vi "ArenaVisualDebugger2017.vi"() -> ()   [LabVIEW 2015, in "MissionControl2017.lvlib" / "DebuggingTools.lvlib"]
uses:
  DebuggingTools.lvlib
  PathfindingSettings.ctl
  MovementSettings.ctl
  PathCostWeights.ctl
  IntermediatePositionGrids.ctl
  <vilib>/Utility/miscctls.llb/LVPoint32TypeDef.ctl
  LocalizationStatus.ctl
  <vilib>/Utility/miscctls.llb/LVBoundsTypeDef.ctl
  Vector.ctl
  Move.ctl
  PathOfMoves.ctl
  Overlord2017.lvlib
  SubVIs - MissionControl2017.lvlib
  TestbenchUtils - Navigation2017.lvlib
  Types - Navigation2017.lvlib
  Navigation2017.lvlib
  SubVIs - Navigation2017.lvlib
panel:
  out "Total Paths Arrived":dbl=484.0
  in  "WaitingForLocalization":bool=TRUE
  in  "Pathfind Turning Radius (m)":dbl(knob)=2.5661842935373853 scale=0.0..4.0
  in  "reset timer":bool
  out "millisecond timer value":u32=9071
  in  "Movement Control Turn Tightness":dbl(slide)=6.226706181197886 scale=1.0..10.0
  out "Right Motor PWM":dbl(graph)
  out "Left Motor PWM":dbl(graph)
  out "Motor PWM XY Graph":cluster{"X":dbl, "Y":dbl}[](graph)
  out "Position at Start of Pathfinding Calculation":T1
  out "Current Localization Status (As Drawn Above)":T1={"x"=4.84866, "y"=1.21078125, "angle"=-2.748893571891069, "valid"=TRUE, "lastUpdatedTime"=858082015.0}
  in  "Debug Mining":bool=TRUE
  in  "Debug Wheel Motors":bool=TRUE
  out "navDebugBotSpin":dbl=-2.748893571891069
  out "y (m)":dbl=0.0221484375
  out "x (m)":dbl=5.26932
  in  "Debug Localization - Mouse":bool=TRUE
  out "Mouse Wheel Sum":dbl=-1.0
  out "Mouse Wheel Delta":i32=-1
  out "Mouse Down Button":u16=1
  out "Mouse Coords":T2={"Horizontal"=286, "Vertical"=3}
  out "Mouse Down Coords":T2={"Horizontal"=343, "Vertical"=164}
  out "CurrMiningRun":i16(slide) scale=0.0..3.0
  out "CurrStage":string
  out "UsedDesperation":bool
  out "SpecifyingEndAngle":bool=TRUE
  out "NextPointIsDestination":bool
  out "CurrNavStage":string
  out "FPS Indicator":bool
  in  "Pathfinding Settings":T3={"Movement Settings"={"Arrival Tolerance (m)"=0.01, "Closeness Threshold (m)"=0.5, "Pit Obstacle Radius (m)"=0.5, "Pit Locations"=[]}, "Dead Zone"=0.85, "Max Moves"=4.0, "Move Segment Length (m)"=0.2, "Path Cost Weights"={"Length Weight"=1.0, "Angle Weight"=0.0, "Angle Error Weight"=1000.0, "Angle Error Threshold"=0.314, "Per Move Penalty"=0.05, "Closeness Weight"=100.0, "Too Short Penalty"=100.0, "Too Short Threshold"=1.5}, "Desperation - Reduction Per Attempt (Ratio)"=0.9, "Desperation - Max Attempts"=1, "Log All Move Points"=TRUE, "Intermediate Position Grids"=[{"x1"=0.0, "x2"=1.75, "resolution"=0.4}, {"x1"=1.75, "x2"=4.5, "resolution"=0.4}]}
  out "Arena Pixel Size":i16[](array[numeric])=[1000, 512]
  out "Arena Control":picture
  # "NOTE: Open and pin\n\nMineOrDumpBlocking.vi\nand\nSetWheelMotorPWM.vi\n\nalongside when debugging."
  # "(Spin robot with arrow keys)"
  # "To toggle localization debugging:\n- Flip this switch <---\n- Set the Project Property -> Conditional Compilation Property\n\"DISCONNECT_LOCALIZATION\" to True or False"
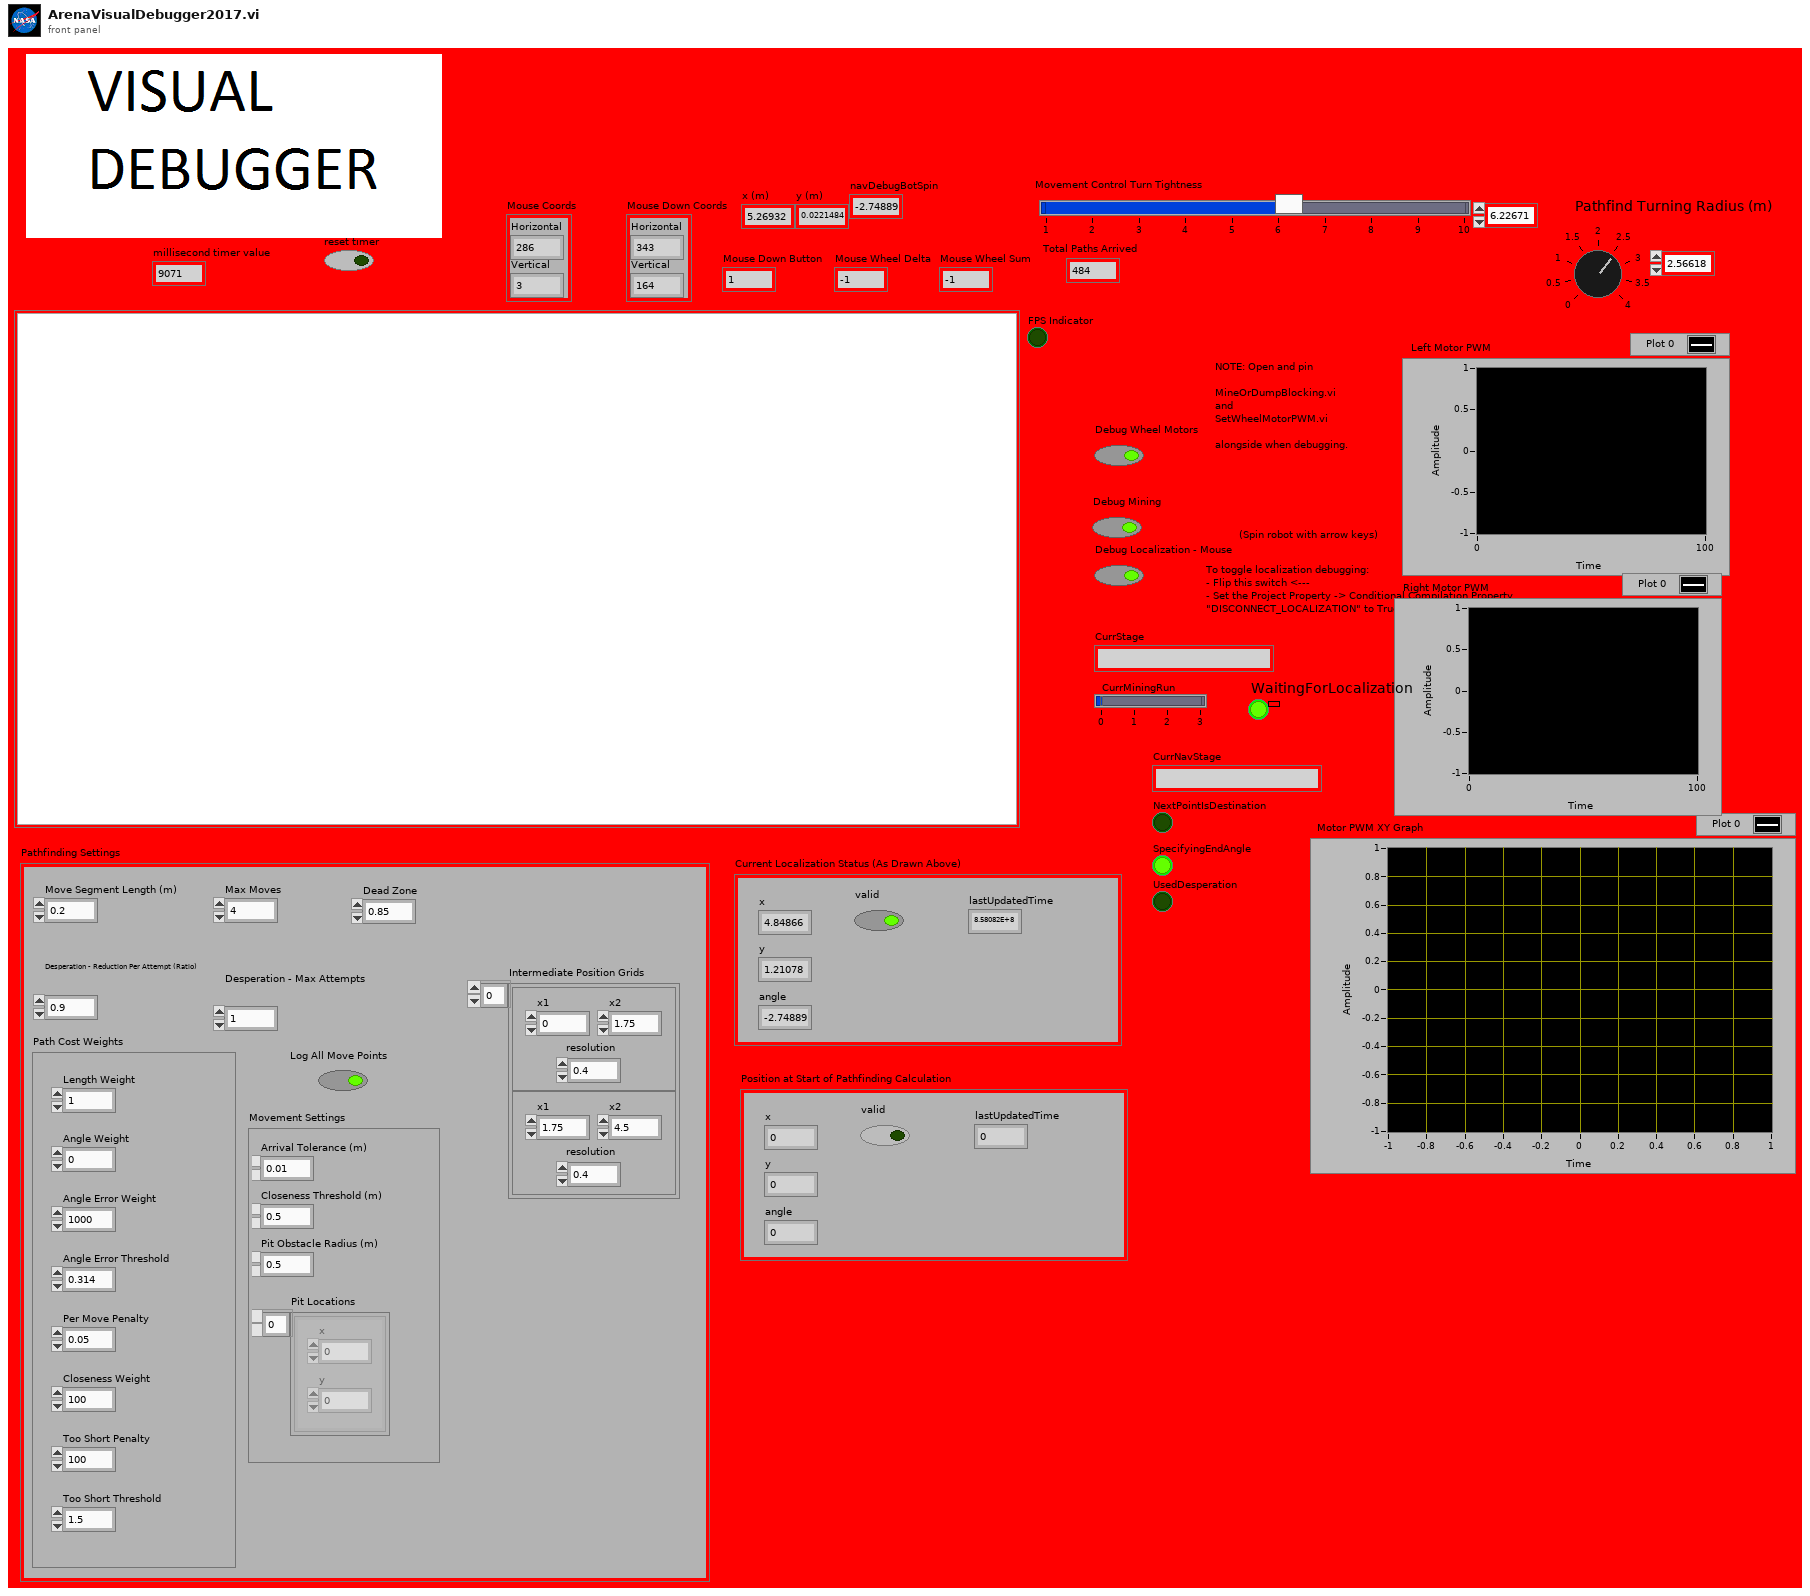
[diagram p1: front panel]
types:
  T1 = typedef "Navigation2017.lvlib/TestbenchUtils - Navigation2017.lvlib/LocalizationStatus.ctl" = cluster{"x":dbl, "y":dbl, "angle":dbl, "valid":bool, "lastUpdatedTime":dbl}
  T2 = typedef "LVPoint32TypeDef.ctl" = cluster{"Horizontal":i32, "Vertical":i32}
  T3 = typedef "Navigation2017.lvlib/Types - Navigation2017.lvlib/PathfindingSettings.ctl" = cluster{"Movement Settings":T4, "Dead Zone":dbl, "Max Moves":dbl, "Move Segment Length (m)":dbl, "Path Cost Weights":T5, "Desperation - Reduction Per Attempt (Ratio)":dbl, "Desperation - Max Attempts":i16, "Log All Move Points":bool, "Intermediate Position Grids":T6}
  T4 = typedef "Navigation2017.lvlib/Types - Navigation2017.lvlib/MovementSettings.ctl" = cluster{"Arrival Tolerance (m)":dbl, "Closeness Threshold (m)":dbl, "Pit Obstacle Radius (m)":dbl, "Pit Locations":cluster{"x":dbl, "y":dbl}[]}
  T5 = typedef "Navigation2017.lvlib/Types - Navigation2017.lvlib/PathCostWeights.ctl" = cluster{"Length Weight":dbl, "Angle Weight":dbl, "Angle Error Weight":dbl, "Angle Error Threshold":dbl, "Per Move Penalty":dbl, "Closeness Weight":dbl, "Too Short Penalty":dbl, "Too Short Threshold":dbl}
  T6 = typedef "Navigation2017.lvlib/Types - Navigation2017.lvlib/IntermediatePositionGrids.ctl" = cluster{"x1":dbl, "x2":dbl, "resolution":dbl}[]
  T7 = typedef "LVBoundsTypeDef.ctl" = cluster{"Width":u32, "Height":u32}
  T8 = typedef "eventvkey.ctl" = enum16{"ASCII", "Enter", "Return", "Shift", "Ctrl", "Alt", "Cmd", "Opt", "Caps", "NumLock", "Clear", "Break", "Up", "Down", "Left", "Right", "Insert", "Delete", "Home", "End", "PageUp", "PageDown", "Escape", "Help", "Pause", "ScrollLock", "F1", "F2", "F3", "F4", "F5", "F6", "F7", "F8", "F9", "F10", "F11", "F12", "F13", "F14", "F15", "F16", "F17", "F18", "F19", "F20", "F21", "F22", "F23", "F24", "Play", "VolumeUp", "VolumeDown", "Mute", "Two Byte Char"}
  T9 = typedef "imagedata.ctl" = cluster{"image type":i32, "image depth":i32, "image":u8[], "mask":u8[], "colors":u32[], "Rectangle":cluster{"left":i16, "top":i16, "right":i16, "bottom":i16}}
  T10 = typedef "Navigation2017.lvlib/Types - Navigation2017.lvlib/Vector.ctl" = cluster{"x":dbl, "y":dbl, "angle":dbl}
  T11 = cluster{"Width":u16, "Style":enum32{"Solid", "Dash", "Dot", "DashDot", "DashDotDot"}}
  T12 = typedef "Navigation2017.lvlib/Types - Navigation2017.lvlib/PathOfMoves.ctl" = cluster{"Dest Angle Error":dbl, "Dest Angle Considered":bool, "Moves":T13[]}
  T13 = typedef "Navigation2017.lvlib/Types - Navigation2017.lvlib/Move.ctl" = cluster{"Did Reach Dest":bool, "Did Collide":bool, "Sum of Angle Changes (rad)":dbl, "Move Length (m)":dbl, "Closeness Sum":dbl, "Positions Along Move":T10[], "Moved Fwd":bool}
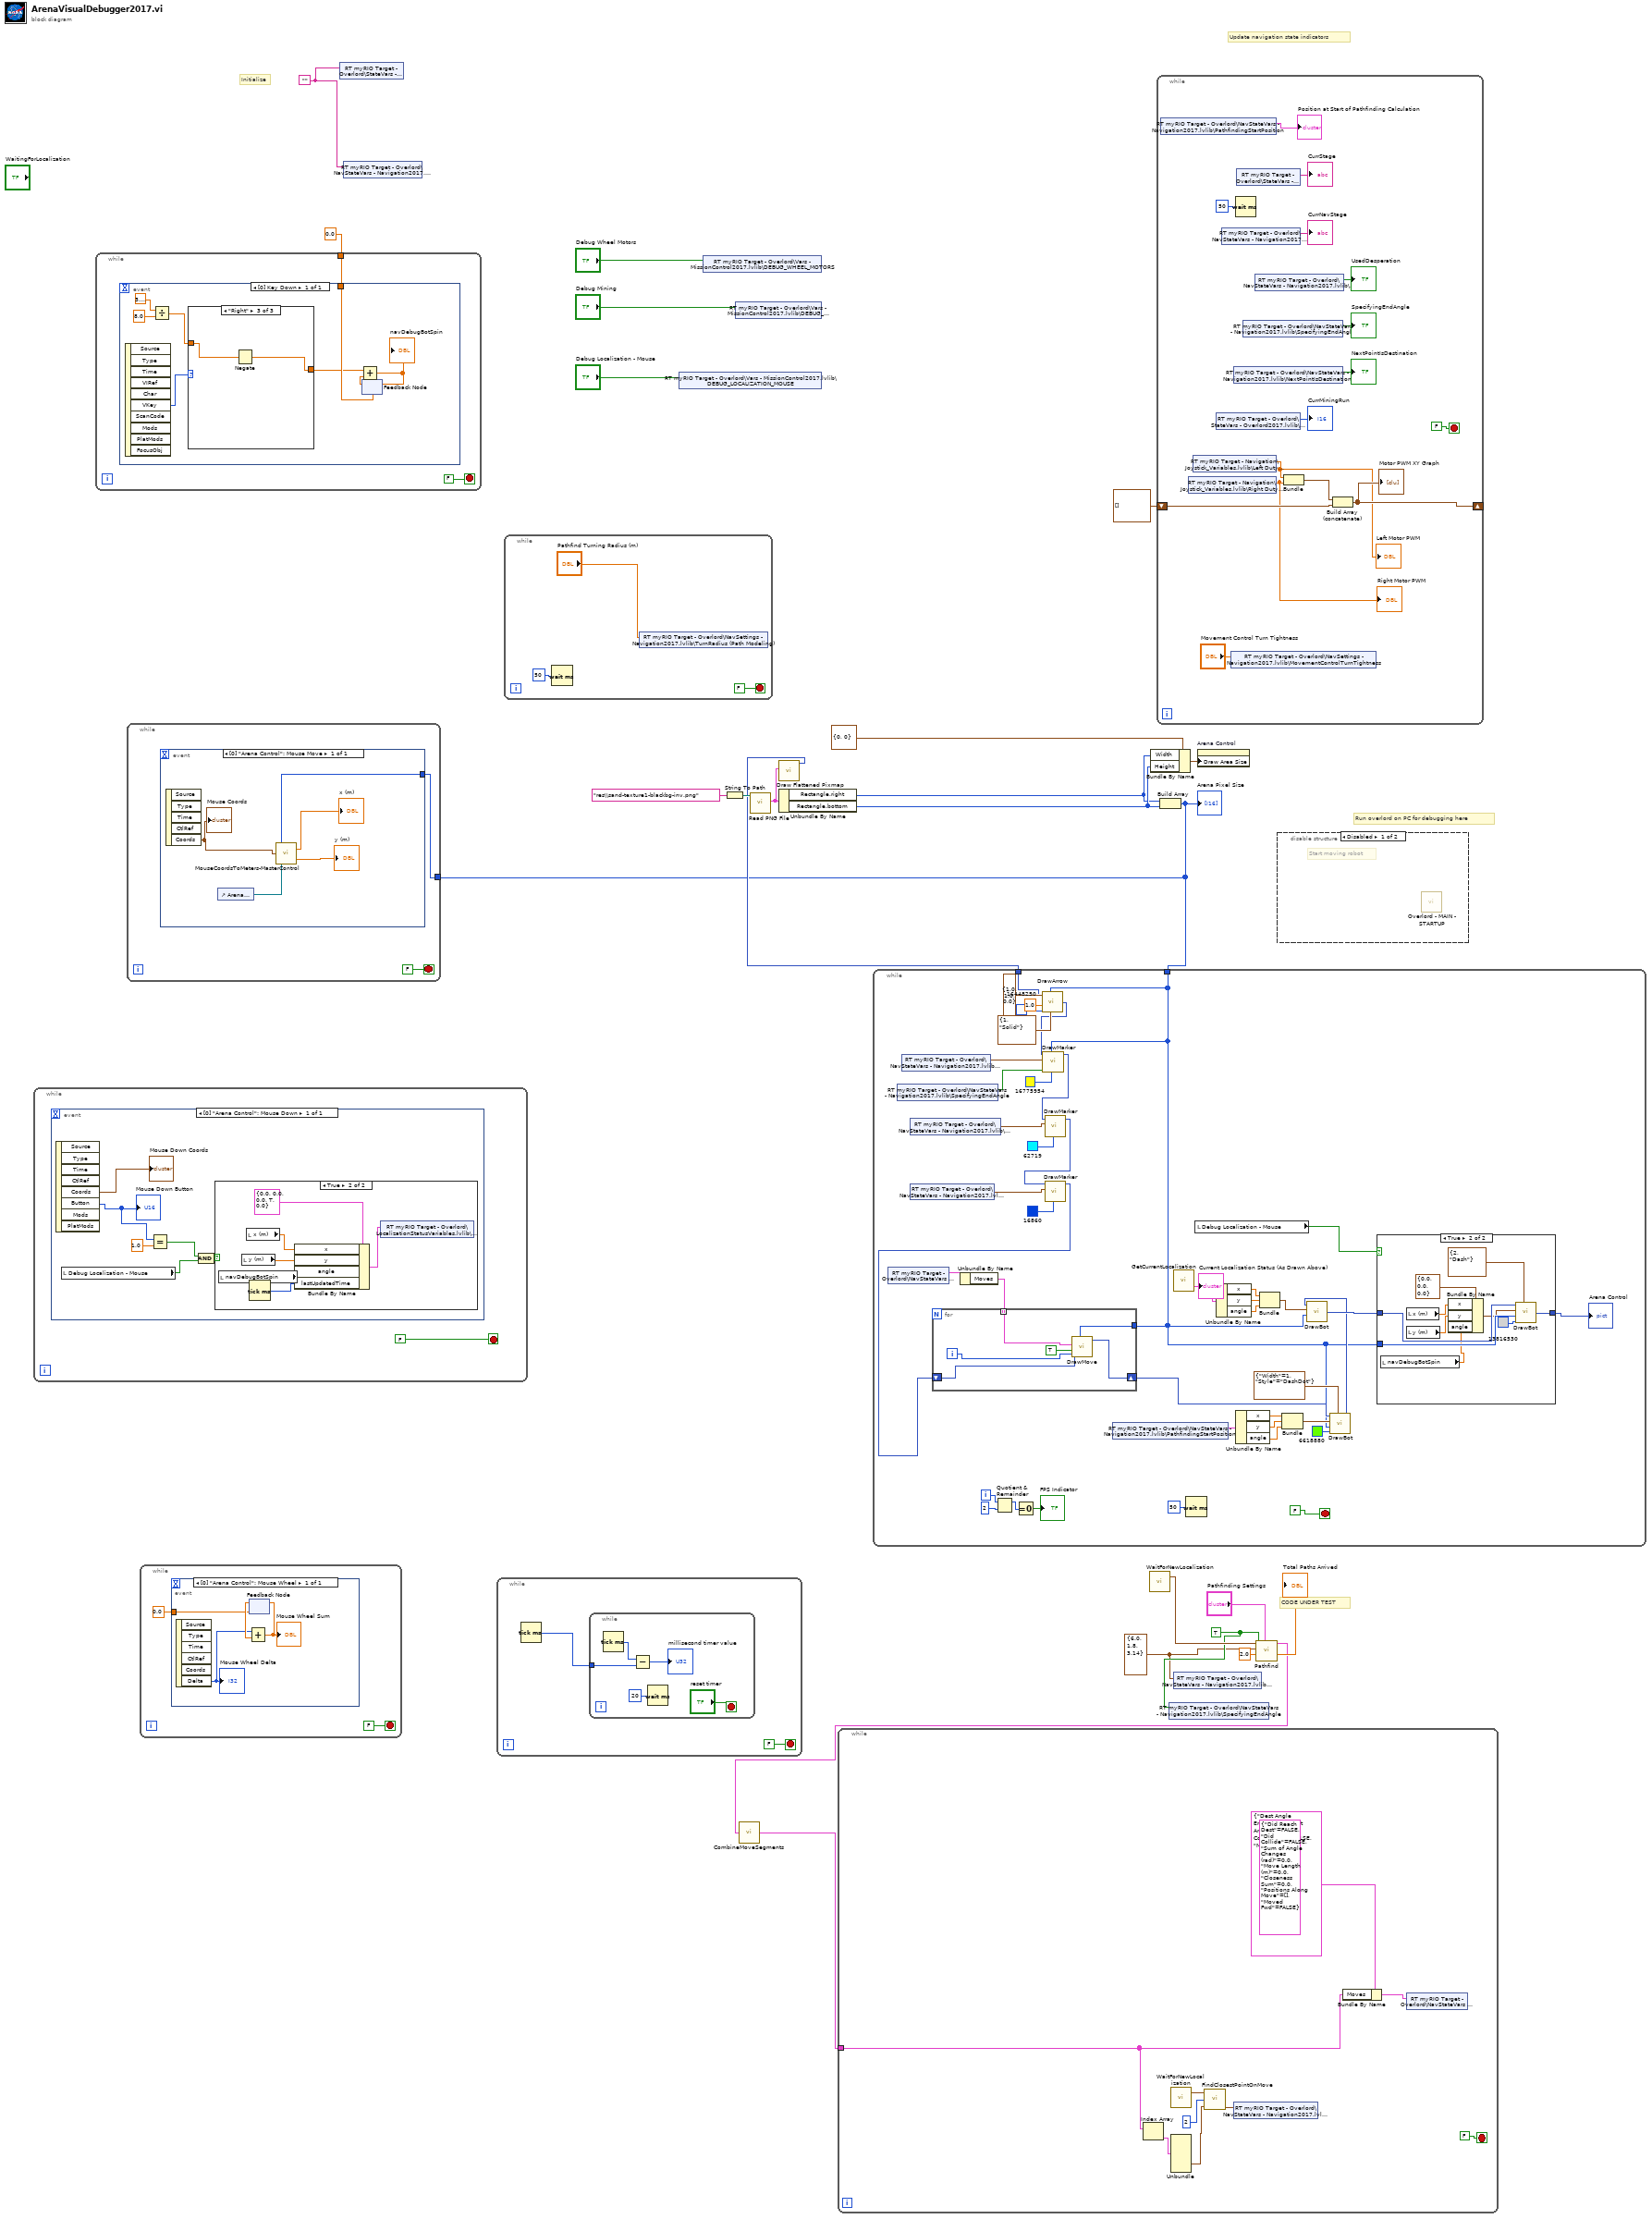
[diagram p0: block diagram]
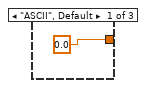
[diagram p3: hidden frame]
diagram:
  w5 = TRUE ("Specified End Angle")
  w4 = cluster{"x":dbl, "y":dbl, "angle":dbl} {"x"=6.0, "y"=1.8, "angle"=3.14} ("Destination")
  w13 = ""
  # "CODE UNDER TEST"
  # "Run overlord on PC for debugging here"
  # "Initialize"
  # "Update navigation state indicators"
  n1 = while {
    stop <- FALSE stop-if-true
    n2 = event shown="[0] \"Arena Control\": Mouse Down" {
      selector: _ -> [_]
      dyn-events: _ -> [_]
      timeout: _ -> [_]
      event "Arena Control": Mouse Down {
        n3 = event-data() -> ("Coords"=→"Mouse Down Coords":T2, "Button"=w28:u16)  [unwired: 1 in, 6 out]
        "Mouse Down Button" <- w28
        n4 = local read "Debug Localization - Mouse"() -> (w27:bool)
        n5 = Equal?(x=w28, y=1.0) -> (x = y?=w26:bool)
        n6 = And(x=w26, y=w27) -> (x .and. y?=w25:bool)
        n7 = case shown="True" w25 {
          frame False {
          }
          frame True {
            n8 = local read "navDebugBotSpin"() -> (w31:dbl)
            n9 = local read "y (m)"() -> (w32:dbl)
            n10 = local read "x (m)"() -> (w33:dbl)
            n11 = Tick Count (ms)() -> (millisecond timer value=w34:u32)
            n12 = Bundle By Name(cluster=T1 {"x"=0.0, "y"=0.0, "angle"=0.0, "valid"=TRUE, "lastUpdatedTime"=0.0} ("Localization Status"), "x"=w33, "y"=w32, "angle"=w31, "lastUpdatedTime"=w34) -> (w35:T1)
            n13 = shared-variable "RT myRIO Target - Overlord\\LocalizationStatusVariables.lvlib\\LocalizationStatus"(w35) -> ()  [unwired: 1 in, 1 out]
          }
        }
      }
    }
  }
  n14 = while {
    tunnel: 0.0 -> [w37]
    stop <- FALSE stop-if-true
    n15 = event shown="[0] Key Down" {
      selector: _ -> [_]
      dyn-events: _ -> [_]
      timeout: _ -> [_]
      tunnel: w37 -> [w43]
      event Key Down {
        n16 = event-data() -> ("VKey"=w46:T8)  [unwired: 1 in, 9 out]
        n17 = Divide(x=3.141592653589793, y=8.0) -> (x/y=w39:dbl)
        n18 = case shown="\"Right\"" w46 {
          tunnel: [0.0 w48 w49] -> w42
          tunnel: w39 -> [_ w48 w50]
          frame "ASCII", Default {
          }
          frame "Left" {
          }
          frame "Right" {
            n19 = Negate(x=w50) -> (-x=w49:dbl)
          }
        }
        n20 = feedback #1(w43) -> (w44:dbl)
        n21 = Add(x=w42, y=w44) -> (x+y=w45:dbl)
        "navDebugBotSpin" <- w45
        n22 = feedback-in #1(w45) -> ()
      }
    }
  }
  n23 = while {
    stop <- FALSE stop-if-true
    n24 = event shown="[0] \"Arena Control\": Mouse Wheel" {
      selector: _ -> [_]
      dyn-events: _ -> [_]
      timeout: _ -> [_]
      tunnel: 0.0 -> [w54]
      event "Arena Control": Mouse Wheel {
        n25 = event-data() -> ("Delta"=w53:i32)  [unwired: 1 in, 5 out]
        "Mouse Wheel Delta" <- w53
        n26 = feedback #2(w54) -> (w55:dbl)
        n27 = Add(x=w53, y=w55) -> (x+y=w56:dbl)
        "Mouse Wheel Sum" <- w56
        n28 = feedback-in #2(w56) -> ()
      }
    }
  }
  n29 = shared-variable "RT myRIO Target - Overlord\\StateVars - Overlord2017.lvlib\\CurrStage"(w13) -> ()  [unwired: 1 in, 1 out]
  n30 = shared-variable "RT myRIO Target - Overlord\\NavStateVars - Navigation2017.lvlib\\CurrNavStage"(w13) -> ()  [unwired: 1 in, 1 out]
  n31 = while {
    stop <- FALSE stop-if-true
    n32 = Tick Count (ms)() -> (millisecond timer value=w58:u32)
    n33 = while {
      tunnel: w58 -> [w60]
      stop <- "reset timer" stop-if-true
      n34 = Tick Count (ms)() -> (millisecond timer value=w61:u32)
      n35 = Subtract(x=w61, y=w60) -> (x-y=→"millisecond timer value":u32)
      n36 = Wait (ms)(milliseconds to wait=u32 20) -> ()  [unwired: 1 out]
    }
  }
  n37 = while {
    stop <- FALSE stop-if-true
    n38 = Wait (ms)(milliseconds to wait=u32 50) -> ()  [unwired: 1 out]
    n39 = shared-variable "RT myRIO Target - Overlord\\NavSettings - Navigation2017.lvlib\\TurnRadius (Path Modeling)"("Pathfind Turning Radius (m)") -> ()  [unwired: 1 in, 1 out]
  }
  n40 = shared-variable "RT myRIO Target - Overlord\\Vars - MissionControl2017.lvlib\\DEBUG_LOCALIZATION_MOUSE"("Debug Localization - Mouse") -> ()  [unwired: 1 in, 1 out]
  n41 = shared-variable "RT myRIO Target - Overlord\\Vars - MissionControl2017.lvlib\\DEBUG_WHEEL_MOTORS"("Debug Wheel Motors") -> ()  [unwired: 1 in, 1 out]
  n42 = String To Path(string="res\\sand-texture1-blackbg-inv.png" ("name or relative path")) -> (path=w22:path)
  n43 = shared-variable "RT myRIO Target - Overlord\\Vars - MissionControl2017.lvlib\\DEBUG_BUCKET"("Debug Mining") -> ()  [unwired: 1 in, 1 out]
  n44 = call <vilib>:"Read PNG File.vi"("path to PNG file"=w22) -> ("image data"=w17:T9)  [unwired: 8 in, 2 out]
  n45 = call <vilib>:"Draw Flattened Pixmap.vi"("image data"=w17) -> ("new picture"=w16:picture)  [unwired: 8 in]
  n46 = Unbundle By Name(w17) -> ("Rectangle.right"=w19:i16, "Rectangle.bottom"=w20:i16)
  n47 = call "WaitForNewLocalization.vi"() -> ("Localization Status Vector"=w6:T10)  [unwired: 1 out]
  n48 = Bundle By Name(cluster=T7 {"Width"=0, "Height"=0} ("Draw Area Size"), "Width"=w19, "Height"=w20) -> (w21:T7)
  n49 = while {
    shift-right: [w70] -> _
    shift-left: cluster{"Double":dbl, "Double":dbl}[] [] -> [w71]
    stop <- FALSE stop-if-true
    n50 = shared-variable "RT myRIO Target - Overlord\\NavStateVars - Navigation2017.lvlib\\PathfindingStartPosition"() -> (→"Position at Start of Pathfinding Calculation":T1)  [unwired: 1 in, 1 out]
    n51 = shared-variable "RT myRIO Target - Navigation\\Joystick_Variables.lvlib\\Right Duty Cycle"() -> (w69:dbl)  [unwired: 1 in, 1 out]
    "Right Motor PWM" <- w69
    n52 = shared-variable "RT myRIO Target - Navigation\\Joystick_Variables.lvlib\\Left Duty Cycle"() -> (w68:dbl)  [unwired: 1 in, 1 out]
    "Left Motor PWM" <- w68
    n53 = shared-variable "RT myRIO Target - Overlord\\StateVars - Overlord2017.lvlib\\CurrMiningRun"() -> (→"CurrMiningRun":i16)  [unwired: 1 in, 1 out]
    n54 = shared-variable "RT myRIO Target - Overlord\\NavStateVars - Navigation2017.lvlib\\CurrNavStage"() -> (→"CurrNavStage":string)  [unwired: 1 in, 1 out]
    n55 = shared-variable "RT myRIO Target - Overlord\\NavSettings - Navigation2017.lvlib\\MovementControlTurnTightness"("Movement Control Turn Tightness") -> ()  [unwired: 1 in, 1 out]
    n56 = shared-variable "RT myRIO Target - Overlord\\NavStateVars - Navigation2017.lvlib\\NextPointIsDestination"() -> (→"NextPointIsDestination":bool)  [unwired: 1 in, 1 out]
    n57 = Wait (ms)(milliseconds to wait=u32 50) -> ()  [unwired: 1 out]
    n58 = shared-variable "RT myRIO Target - Overlord\\StateVars - Overlord2017.lvlib\\CurrStage"() -> (→"CurrStage":string)  [unwired: 1 in, 1 out]
    n59 = shared-variable "RT myRIO Target - Overlord\\NavStateVars - Navigation2017.lvlib\\SpecifyingEndAngle"() -> (→"SpecifyingEndAngle":bool)  [unwired: 1 in, 1 out]
    n60 = shared-variable "RT myRIO Target - Overlord\\NavStateVars - Navigation2017.lvlib\\UsedDesperation"() -> (→"UsedDesperation":bool)  [unwired: 1 in, 1 out]
    n61 = Bundle("Double"=w68, "Double"=w69) -> (w72:cluster{"Double":dbl, "Double":dbl})  [unwired: 1 in]
    n62 = Build Array (concatenate)(w72, w71) -> (w70:cluster{"Double":dbl, "Double":dbl}[])
    "Motor PWM XY Graph" <- w70
  }
  n63 = Build Array(w19, w20) -> (w14:i16[])
  "Arena Pixel Size" <- w14
  n64 = while {
    tunnel: w14 -> [w82]
    stop <- FALSE stop-if-true
    n65 = event shown="[0] \"Arena Control\": Mouse Move" {
      selector: _ -> [_]
      dyn-events: _ -> [_]
      timeout: _ -> [_]
      tunnel: w82 -> [w87]
      event "Arena Control": Mouse Move {
        n66 = event-data() -> ("Coords"=w88:T2)  [unwired: 1 in, 4 out]
        "Mouse Coords" <- w88
        n67 = control-ref of="Arena Control"() -> (w86:refnum<vi>)
        n68 = call "MouseCoordsToMeters-MasterControl.vi"("Picture Control Ref"=w86, "Mouse Pos"=w88, "Arena Pixel Dim"=w87) -> ("y (m)"=→"y (m)":dbl, "x (m)"=→"x (m)":dbl)
      }
    }
  }
  n69 = while {
    tunnel: w16 -> [w91]
    tunnel: w14 -> [w90]
    i -> [w129]
    stop <- FALSE stop-if-true
    n70 = shared-variable "RT myRIO Target - Overlord\\NavStateVars - Navigation2017.lvlib\\CurrPath"() -> (w117:T12)  [unwired: 1 in, 1 out]
    n71 = shared-variable "RT myRIO Target - Overlord\\NavStateVars - Navigation2017.lvlib\\SpecifyingEndAngle"() -> (w109:bool)  [unwired: 1 in, 1 out]
    n72 = shared-variable "RT myRIO Target - Overlord\\NavStateVars - Navigation2017.lvlib\\DestinationPoint"() -> (w110:T10)  [unwired: 1 in, 1 out]
    n73 = shared-variable "RT myRIO Target - Overlord\\NavStateVars - Navigation2017.lvlib\\NextPointOnPath"() -> (w111:T10)  [unwired: 1 in, 1 out]
    n74 = shared-variable "RT myRIO Target - Overlord\\NavStateVars - Navigation2017.lvlib\\CurrPosOnPath"() -> (w99:T10)  [unwired: 1 in, 1 out]
    n75 = Unbundle By Name(w117) -> ("Moves"=w116:T13[])
    n76 = Quotient & Remainder(x=w129, y=2) -> (x-y*floor(x/y)=w120:i32)  [unwired: 1 out]
    n77 = Equal To 0?(x=w120) -> (x = 0?=→"FPS Indicator":bool)
    n78 = call "DrawArrow.vi"("Pen Style"=T11 {"Width"=1, "Style"=enum."Solid"}, "Arena Pixel Dim"=w90, "Color"=u32 16448250, "Length (m)"=1.0, "Vector (m)"=T10 {"x"=1.0, "y"=1.0, "angle"=0.0}, "picture"=w91) -> ("new picture"=w89:picture)
    n79 = call "DrawMarker.vi"("color(black)"=u32 16775954, "Arena Pixel Dim"=w90, "Draw An Arrow"=w109, "Cluster"=w110, "picture in"=w89) -> ("new picture"=w115:picture)  [unwired: 6 in]
    n80 = call "DrawMarker.vi"("color(black)"=u32 62719, "Cluster"=w111, "picture in"=w115) -> ("new picture"=w97:picture)  [unwired: 8 in]
    n81 = call "DrawMarker.vi"("color(black)"=u32 16860, "Cluster"=w99, "picture in"=w97) -> ("new picture"=w96:picture)  [unwired: 8 in]
    n82 = for {
      tunnel: w90 -> [w134]
      shift-right: [w135] -> w108
      shift-left: w96 -> [w136]
      tunnel: w116 -> [w132] mode=indexing
      i -> [w131]
      n83 = call "DrawMove.vi"("Arena Pixel Dim"=w134, "Move Number (optional)"=w131, "Show Vectors?"=TRUE, "Move"=w132, "picture in"=w136) -> ("picture out"=w135:picture)  [unwired: 3 in]
    }
    n84 = shared-variable "RT myRIO Target - Overlord\\NavStateVars - Navigation2017.lvlib\\PathfindingStartPosition"() -> (w103:T1)  [unwired: 1 in, 1 out]
    n85 = call "GetCurrentLocalization.vi"() -> ("Current Localization Status"=w122:T1)  [unwired: 1 out]
    "Current Localization Status (As Drawn Above)" <- w122
    n86 = Wait (ms)(milliseconds to wait=u32 50) -> ()  [unwired: 1 out]
    n87 = local read "Debug Localization - Mouse"() -> (w112:bool)
    n88 = Unbundle By Name(w122) -> ("x"=w125:dbl, "y"=w124:dbl, "angle"=w123:dbl)
    n89 = Unbundle By Name(w103) -> ("x"=w102:dbl, "y"=w101:dbl, "angle"=w100:dbl)
    n90 = Bundle("x"=w125, "y"=w124, "angle"=w123) -> (w121:cluster{"x":dbl, "y":dbl, "angle":dbl})  [unwired: 1 in]
    n91 = Bundle("x"=w102, "y"=w101, "angle"=w100) -> (w104:cluster{"x":dbl, "y":dbl, "angle":dbl})  [unwired: 1 in]
    n92 = call "DrawBot.vi"("picture in"=w108, "bot pos vector"=w104, "Arena Pixel Size"=w90, "bot color"=u32 6618880, "pen"=T11 {"Width"=1, "Style"=enum."DashDot"}) -> ("picture out"=w107:picture)
    n93 = call "DrawBot.vi"("picture in"=w107, "bot pos vector"=w121, "Arena Pixel Size"=w90) -> ("picture out"=w119:picture)  [unwired: 2 in]
    n94 = case shown="True" w112 {
      tunnel: w119 -> [w137 w147]
      tunnel: [w137 w146] -> w118
      tunnel: w90 -> [_ w143]
      frame False {
      }
      frame True {
        n95 = local read "navDebugBotSpin"() -> (w138:dbl)
        n96 = local read "x (m)"() -> (w140:dbl)
        n97 = local read "y (m)"() -> (w141:dbl)
        n98 = Bundle By Name(cluster=T10 {"x"=0.0, "y"=0.0, "angle"=0.0} ("Vector"), "x"=w140, "y"=w141, "angle"=w138) -> (w142:T10)
        n99 = call "DrawBot.vi"("picture in"=w147, "bot pos vector"=w142, "Arena Pixel Size"=w143, "bot color"=u32 13816530, "pen"=T11 {"Width"=2, "Style"=enum."Dash"}) -> ("picture out"=w146:picture)
      }
    }
    "Arena Control" <- w118
  }
  n100 = shared-variable "RT myRIO Target - Overlord\\NavStateVars - Navigation2017.lvlib\\SpecifyingEndAngle"(w5) -> ()  [unwired: 1 in, 1 out]
  n101 = shared-variable "RT myRIO Target - Overlord\\NavStateVars - Navigation2017.lvlib\\DestinationPoint"(w4) -> ()  [unwired: 1 in, 1 out]
  n102 = property on="Arena Control" class="Pict"("Draw Area Size"=w21) -> ()  [unwired: 2 in, 2 out]
  n103 = call "Pathfind.vi"("Pathfinding Settings"="Pathfinding Settings", "Specified End Angle"=w5, "Turn Radius (m)"=2.0, "Destination"=w4, "Start Vector"=w6) -> ("Total Paths Arrived"=→"Total Paths Arrived":dbl, "Best Path"=w2:T12)  [unwired: 3 out]
  n104 = call "CombineMoveSegments.vi"("Path"=w2) -> ("Combined Moves (Discarding Metadata Save Moved Fwd)"=w1:T13[])
  n105 = while {
    tunnel: w1 -> [w149]
    stop <- FALSE stop-if-true
    (unwired) T13 {"Did Reach Dest"=FALSE, "Did Collide"=FALSE, "Sum of Angle Changes (rad)"=0.0, "Move Length (m)"=0.0, "Closeness Sum"=0.0, "Positions Along Move"=[], "Moved Fwd"=FALSE} ("Move")
    n106 = Index Array(array=w149) -> (element=w154:T13)  [unwired: 1 in]
    n107 = call "WaitForNewLocalization.vi"() -> ("Localization Status Vector"=w153:T10)  [unwired: 1 out]
    n108 = Unbundle(w154) -> ("Positions Along Move"=w148:T10[])  [unwired: 6 out]
    n109 = call "FindClosestPointOnMove.vi"("Current Robot Position"=w153, "Start Index"=2, "Move Positions"=w148) -> ("Closest Vector"=w155:T10)  [unwired: 3 out]
    n110 = shared-variable "RT myRIO Target - Overlord\\NavStateVars - Navigation2017.lvlib\\CurrPosOnPath"(w155) -> ()  [unwired: 1 in, 1 out]
    n111 = Bundle By Name(cluster=T12 {"Dest Angle Error"=0.0, "Dest Angle Considered"=FALSE, "Moves"=[]} ("Path"), "Moves"=w149) -> (w150:T12)
    n112 = shared-variable "RT myRIO Target - Overlord\\NavStateVars - Navigation2017.lvlib\\CurrPath"(w150) -> ()  [unwired: 1 in, 1 out]
  }
  n113 = disable-structure shown="Disabled" {
    frame Disabled {
      # "Start moving robot"
      n114 = call "Overlord - MAIN - STARTUP.vi"() -> ("Pathfinding Settings"=w157:T3)
    }
    frame Enabled {
    }
  }
